vi "get_cutoff_pixels.vi"(8 "error in (no error)":errorcluster, 11 "DL090211FrameImageAssembler in":refnum<class "ImageAssemblerDL090211Frame.lvclass">) -> (0 "error out":errorcluster, 1 "right cut-off":i32, 2 "left cut-off":i32, 3 "DL090211FrameImageAssembler out":refnum<class "ImageAssemblerDL090211Frame.lvclass">, 4 "total cut-off":i32, 5 "total pixels per line":i32)   [LabVIEW 2010, in "ImageAssemblerDL090211Frame.lvclass"]
uses:
  ImageAssemblerDL090211Frame.lvclass
  ImageAssemblerDL090211Frame.lvclass/ImageAssemblerDL090211Frame.ctl
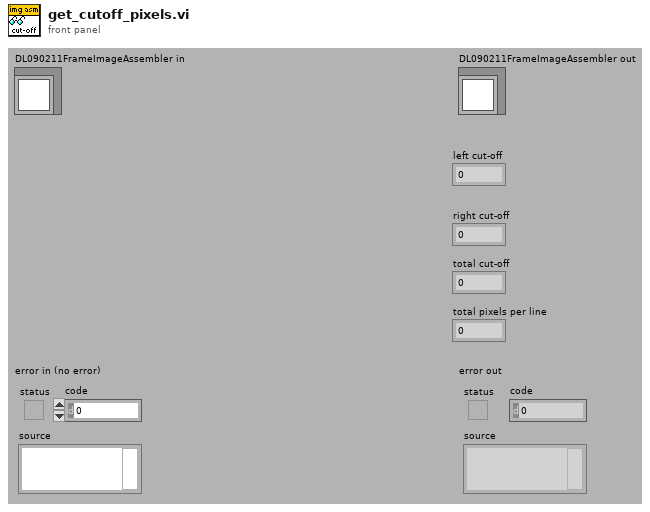
[diagram p1: front panel]
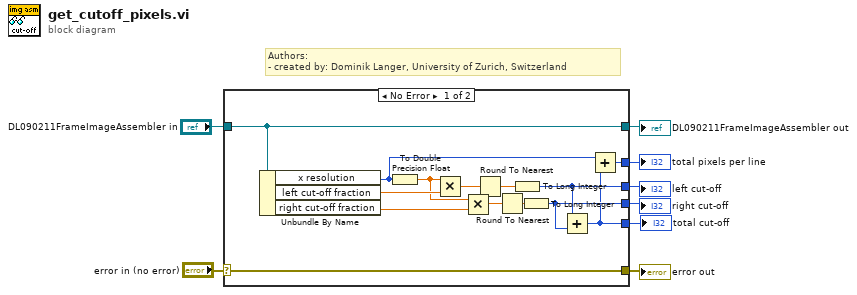
[diagram p0: block diagram]
diagram:
  # "Authors: \n- created by: Dominik Langer, University of Zurich, Switzerland"
  n1 = case shown="No Error" "error in (no error)" {
    selector: "error in (no error)" -> [w22 w24]
    tunnel: [w22 w24] -> w7
    tunnel: [w21 w23] -> w5
    tunnel: "DL090211FrameImageAssembler in" -> [w21 w23]
    tunnel: [w13 _] -> w4
    tunnel: [w12 _] -> w3
    tunnel: [w11 _] -> w2
    tunnel: [w9 _] -> w1
    frame No Error {
      n2 = Unbundle By Name(w21) -> ("x resolution"=w10:i32, "left cut-off fraction"=w20:dbl, "right cut-off fraction"=w18:dbl)
      n3 = To Double Precision Float(number=w10) -> (double precision float=w19:dbl)
      n4 = Multiply(x=w19, y=w20) -> (x*y=w17:dbl)
      n5 = Multiply(x=w19, y=w18) -> (x*y=w14:dbl)
      n6 = Round To Nearest(number=w17) -> (nearest integer value=w16:dbl)
      n7 = Round To Nearest(number=w14) -> (nearest integer value=w15:dbl)
      n8 = To Long Integer(number=w16) -> (32bit integer=w13:i32)
      n9 = To Long Integer(number=w15) -> (32bit integer=w12:i32)
      n10 = Add(x=w13, y=w12) -> (x+y=w11:i32)
      n11 = Add(x=w10, y=w11) -> (x+y=w9:i32)
    }
    frame Error {
    }
  }
  "error out" <- w7
  "DL090211FrameImageAssembler out" <- w5
  "left cut-off" <- w4
  "right cut-off" <- w3
  "total cut-off" <- w2
  "total pixels per line" <- w1
